vi "FindSession.vi"(0 "Session Handle in":T1, 5 "Session  Name ()":string, 9 "Get new if not exist?":bool, 11 "error in (no error)":errorcluster) -> (4 "Session Handle out":T1, 6 "Session Valid?":bool, 15 "error out":errorcluster)   [LabVIEW 2019, in "SmartScopeDriver.lvclass"]
doc: "Checks if a Session has already been created and returns the session handle or creates a new session."
uses:
  SmartScopeDriver.lvclass
  Typedefs/Session Handle.ctl
  C:/Program Files (x86)/National Instruments/LabVIEW 2019/user.lib/_Session Fwk/Session - Root.lvclass
  <userlib>/_Session Fwk/Session - Root.lvclass
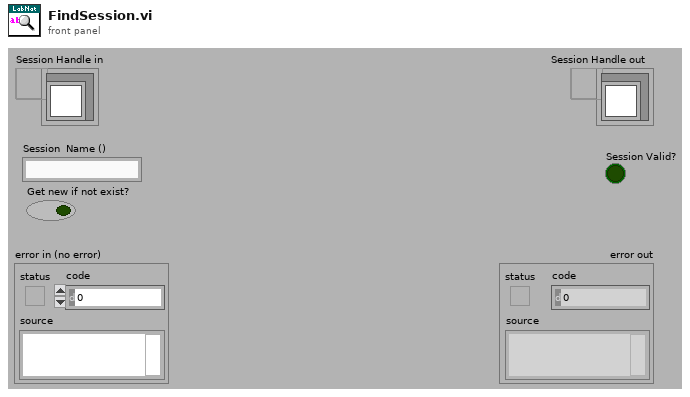
[diagram p1: front panel]
types:
  T1 = typedef "SmartScopeDriver.lvclass/Session Handle.ctl" = refnum<data-value>
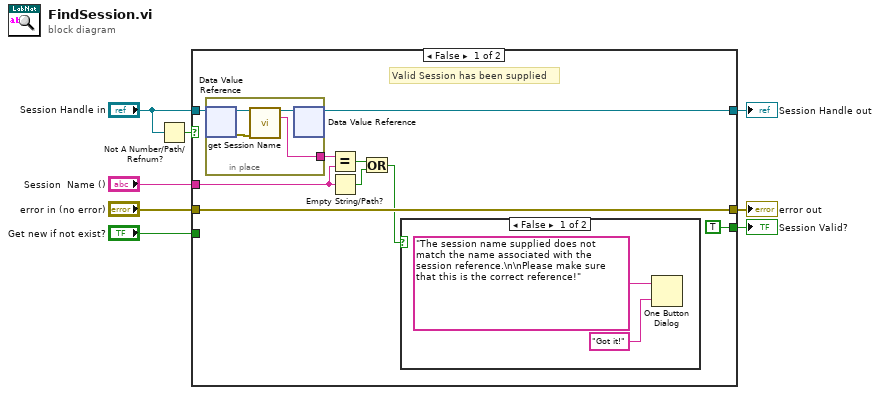
[diagram p0: block diagram]
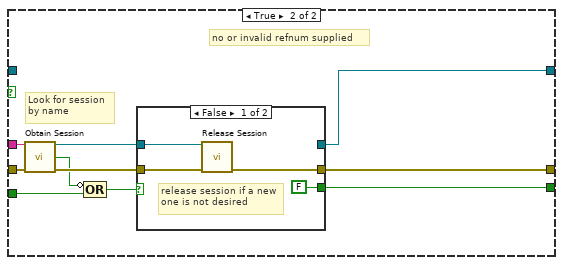
[diagram p3: hidden frame]
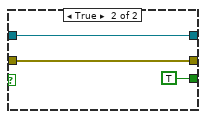
[diagram p4: hidden frame]
diagram:
  n1 = Not A Number/Path/Refnum?(number/path/refnum="Session Handle in") -> (NaN/Path/Refnum?=w8:bool)
  n2 = case shown="False" w8 {
    tunnel: [w14 w30] -> w4
    tunnel: "Session  Name ()" -> [w11 w27]
    tunnel: "Session Handle in" -> [w15 _]
    tunnel: "error in (no error)" -> [w17 w29]
    tunnel: [w17 w31] -> w6
    tunnel: [TRUE ("Session Valid?") w28] -> w3
    tunnel: "Get new if not exist?" -> [_ w26]
    frame False {
      # "Valid Session has been supplied"
      n3 = in-place {
        in-place-border: [w18] -> w13
        n4 = in-place-dvr #1(w15) -> (w21:refnum<class "SmartScopeDriver.lvclass">, w19:errorcluster)
        n5 = call <userlib>:"get Session Name.vi"("OBJ - Session in"=w21, "error in (no error)"=w19) -> ("OBJ - Session out"=w20:refnum<class "SmartScopeDriver.lvclass">, "Session Name"=w18:string)  [unwired: 11 in, 1 out]
        n6 = in-place-dvr #1(w20) -> (w14:T1)  [unwired: 1 out]
      }
      n7 = Equal?(x=w13, y=w11) -> (x = y?=w12:bool)
      n8 = Empty String/Path?(string/path=w11) -> (empty?=w9:bool)
      n9 = Or(x=w12, y=w9) -> (x .or. y?=w10:bool)
      n10 = case shown="False" w10 {
        frame False {
          n11 = One Button Dialog(message="The session name supplied does not match the name associated with the session reference.\n\nPlease make sure that this is the correct reference!", button name ("OK")="Got it!") -> ()  [unwired: 1 out]
        }
        frame True {
        }
      }
    }
    frame True {
      # "Look for session\nby name"
      # "no or invalid refnum supplied"
      n12 = call "Obtain Session.vi"("Session  Name ()"=w27, "error in (no error)"=w29) -> ("Session Handle"=w33:T1, "created new?"=w25:bool, "error out"=w32:errorcluster)  [unwired: 11 in]
      n13 = Compound Arithmetic op=OR(invert w25, w26) -> (w24:bool)
      n14 = case shown="False" w24 {
        tunnel: w33 -> [w37 w39]
        tunnel: w32 -> [w36 w40]
        tunnel: [w35 w40] -> w31
        tunnel: [_ w39] -> w30
        tunnel: [FALSE ("Session Acquired") TRUE ("Session Acquired?")] -> w28
        frame False {
          # "release session if a new\none is not desired"
          n15 = call "Release Session.vi"("Session Handle"=w37, "error in (no error)"=w36) -> ("error out"=w35:errorcluster)  [unwired: 13 in]
        }
        frame True {
        }
      }
    }
  }
  "Session Handle out" <- w4
  "error out" <- w6
  "Session Valid?" <- w3
